vi "TEST ATAN2 and joystick functions.vi"() -> ()   [LabVIEW 2023]
panel:
  out "Array":T1(array[cluster]) {"Jx" format="%#.4f"; "Jy" format="%#.4f"; "R" format="%#.4f"; "theta (rad)" format="%#.4f"}
  in  "Joystick":cluster{"Jx":dbl, "Jy":dbl, "Jr":dbl}[](array[cluster])
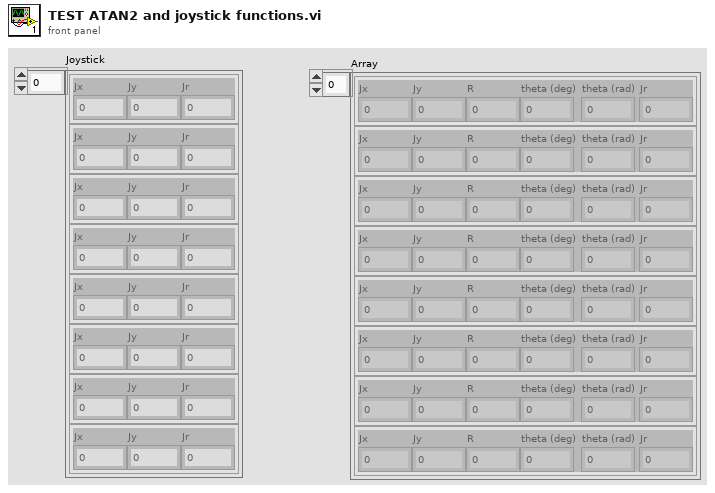
[diagram p1: front panel]
types:
  T1 = cluster{"Jx":dbl, "Jy":dbl, "R":dbl, "theta (deg)":dbl, "theta (rad)":dbl, "Jr":dbl}[]
  T2 = cluster{"Jx":dbl, "Jy":dbl, "R":dbl, "theta (deg)":dbl, "theta (rad)":dbl, "Jr":dbl}
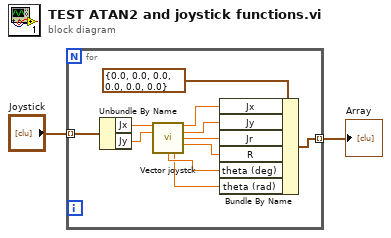
[diagram p0: block diagram]
diagram:
  n1 = for {
    tunnel: "Joystick" -> [w13] mode=indexing
    tunnel: [w9] -> w1 mode=indexing
    n2 = Unbundle By Name(w13) -> ("Jx"=w12:dbl, "Jy"=w11:dbl)
    n3 = call "Vector joystck.vi"("Jx input"=w12, "Jy input"=w11) -> ("Jx"=w5:dbl, "Jy"=w4:dbl, "Jr"=w8:dbl, "R"=w7:dbl, "theta (deg)"=w6:dbl, "theta (rad)"=w3:dbl)  [unwired: 8 in]
    n4 = Bundle By Name(cluster=T2 {"Jx"=0.0, "Jy"=0.0, "R"=0.0, "theta (deg)"=0.0, "theta (rad)"=0.0, "Jr"=0.0} ("Cluster"), "Jx"=w5, "Jy"=w4, "Jr"=w8, "R"=w7, "theta (deg)"=w6, "theta (rad)"=w3) -> (w9:T2)
  }
  "Array" <- w1
